vi "Write Group.vi"(8 "error in (no error)":errorcluster, 10 "Group":string="Untitled", 11 "Acquired Result in":refnum<class "Acquired Result.lvclass">) -> (0 "error out":errorcluster, 3 "Acquired Result out":refnum<class "Acquired Result.lvclass">)   [LabVIEW 2019, in "Acquired Result.lvclass"]
uses:
  Acquired Result.lvclass
  Acquired Result.lvclass/Acquired Result.ctl
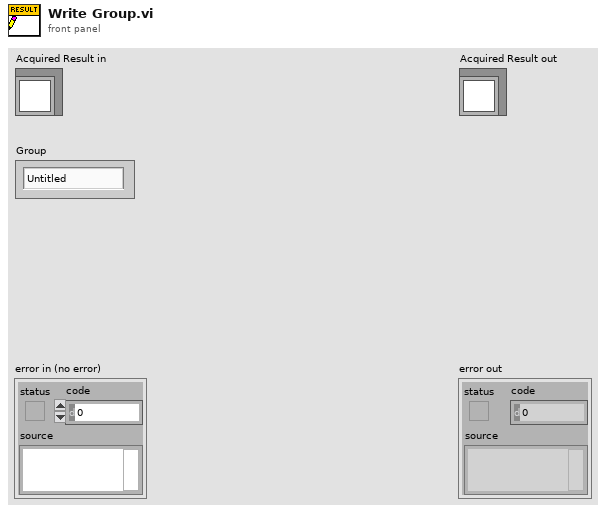
[diagram p1: front panel]
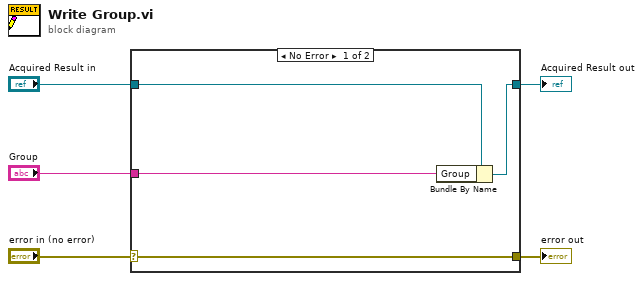
[diagram p0: block diagram]
diagram:
  n1 = case shown="No Error" "error in (no error)" {
    selector: "error in (no error)" -> [w9 w10]
    tunnel: [w9 w10] -> w4
    tunnel: [w7 w11] -> w2
    tunnel: "Acquired Result in" -> [w8 w11]
    tunnel: "Group" -> [w6 _]
    frame No Error {
      n2 = Bundle By Name(cluster=w8, "Group"=w6) -> (w7:refnum<class "Acquired Result.lvclass">)
    }
    frame Error {
    }
  }
  "error out" <- w4
  "Acquired Result out" <- w2
